vi "Perform Action.vi"(8 "error in":errorcluster, 10 "Input":variant, 11 "Red-y Read Write CFG in":refnum<class "Red-y Read Write CFG.lvclass">) -> (0 "error out":errorcluster, 2 "Output":variant, 3 "Red-y Read Write CFG out":refnum<class "Red-y Read Write CFG.lvclass">)   [LabVIEW 2023, in "Red-y Read Write CFG.lvclass"]
uses:
  Red-y Read Write CFG.lvclass
  Red-y Read Write CFG.lvclass/Red-y Read Write CFG.ctl
  Voegtlin_NI_SMART_Modbus_Drivers/Low Level Driver/Modbus Write U8.vi
  Voegtlin_NI_SMART_Modbus_Drivers/Low Level Driver/Modbus Write U16.vi
  Voegtlin_NI_SMART_Modbus_Drivers/Low Level Driver/Modbus Write U32.vi
  Voegtlin_NI_SMART_Modbus_Drivers/Low Level Driver/Modbus Write SGL.vi
  Voegtlin_NI_SMART_Modbus_Drivers/Low Level Driver/Modbus Write STR50.vi
  Voegtlin_NI_SMART_Modbus_Drivers/Low Level Driver/Modbus Read U8.vi
  Voegtlin_NI_SMART_Modbus_Drivers/Low Level Driver/Modbus Read U16.vi
  Voegtlin_NI_SMART_Modbus_Drivers/Low Level Driver/Modbus Read U32.vi
  Voegtlin_NI_SMART_Modbus_Drivers/Low Level Driver/Modbus Read SGL.vi
  Voegtlin_NI_SMART_Modbus_Drivers/Low Level Driver/Modbus Read STR50.vi
  <userlib>/_OpenG.lib/lvdata/lvdata.llb/openg_variant.lvlib
  Voegtlin_NI_SMART_Modbus_Drivers/Voegtlin_NI_SMART_Modbus_Drivers.lvlib
  Read Write PE Input.ctl
  <vilib>/ErrorRing/Error Ring.xnode
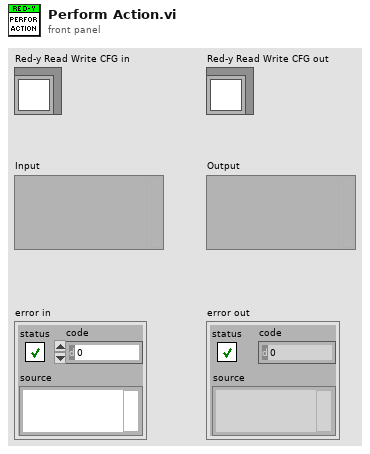
[diagram p1: front panel]
types:
  T1 = typedef "Read Write PE Input.ctl" = cluster{"Action":enum16{"Write", "Read"}, "Register Start Address":u16, "Data (Type)":variant}
  T2 = typedef "openg_variant.lvlib/Type Descriptor Enumeration__ogtk.ctl" = enum8{"<Null>", "I8", "I16", "I32", "I64", "U8", "U16", "U32", "U64", "SGL", "DBL", "EXT", "CSG", "CDB", "CXT", "0x0F", "0x10", "0x11", "0x12", "0x13", "0x14", "Enum U8", "Enum U16", "Enum U32", "Enum U64", "SGL PQ", "DBL PQ", "EXT PQ", "CSG PQ", "CDB PQ", "CXT PQ", "0x1F", "0x20", "Boolean", "0x22", "0x23", "0x24", "0x25", "0x26", "0x27", "0x28", "0x29", "0x2A", "0x2B", "0x2C", "0x2D", "0x2E", "0x2F", "String", "0x31", "Path", "Pict", "0x34", "0x35", "0x36", "DAQ", "0x38", "0x39", "0x3A", "0x3B", "0x3C", "0x3D", "0x3E", "0x3F", "Array", "0x41", "0x42", "0x43", "0x44", "0x45", "0x46", "0x47", "0x48", "0x49", "0x4A", "0x4B", "0x4C", "0x4D", "0x4E", "0x4F", "Cluster", "0x51", "0x52", "Variant", "Waveform", "0x55", "0x56", "0x57", "0x58", "0x59", "0x5A", "0x5B", "0x5C", "0x5D", "0x5E", "Fixed Point", "0x60", "0x61", "0x62", "0x63", "0x64", "0x65", "0x66", "0x67", "0x68", "0x69", "0x6A", "0x6B", "0x6C", "0x6D", "0x6E", "0x6F", "Refnum", "0x71", "0x72", "Set Collection", "Map Collection"}
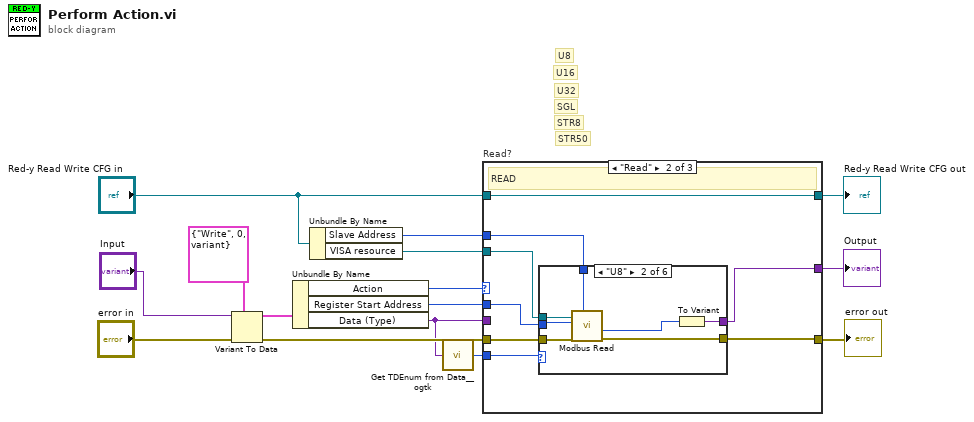
[diagram p0: block diagram]
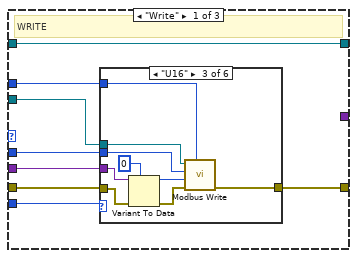
[diagram p2: hidden frame]
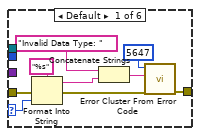
[diagram p3: hidden frame]
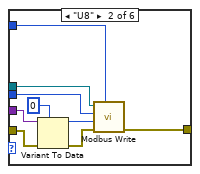
[diagram p4: hidden frame]
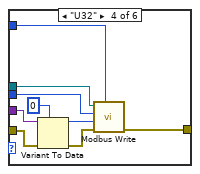
[diagram p5: hidden frame]
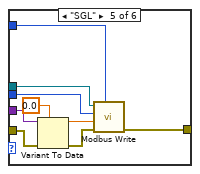
[diagram p6: hidden frame]
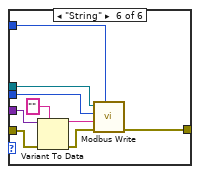
[diagram p7: hidden frame]
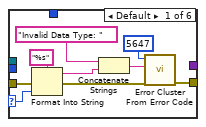
[diagram p8: hidden frame]
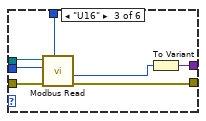
[diagram p9: hidden frame]
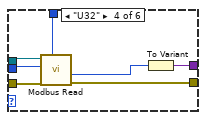
[diagram p10: hidden frame]
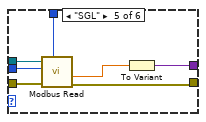
[diagram p11: hidden frame]
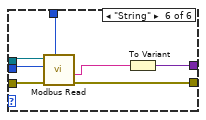
[diagram p12: hidden frame]
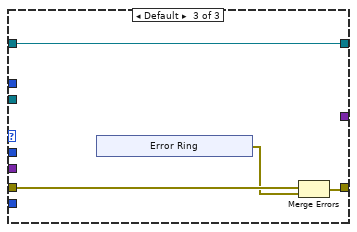
[diagram p13: hidden frame]
diagram:
  # "STR50"
  # "STR8"
  # "SGL"
  # "U32"
  # "U16"
  # "U8"
  n1 = Variant To Data(error in="error in", type=T1 {"Action"=enum."Write", "Register Start Address"=0, "Data (Type)"=variant}, Variant="Input") -> (data=w8:T1, error out=w11:errorcluster)
  n2 = Unbundle By Name(w8) -> ("Action"=w1:enum16{"Write", "Read"}, "Register Start Address"=w3:u16, "Data (Type)"=w2:variant)
  n3 = Unbundle By Name("Red-y Read Write CFG in") -> ("Slave Address"=w6:u8, "VISA resource"=w5:refnum<visa-resource-name>)
  n4 = call <userlib>:"Get TDEnum from Data__ogtk.vi"("Data"=w2) -> ("Type Descriptor Enumeration"=w4:T2)  [unwired: 4 in]
  n5 = case "Read?" shown="\"Read\"" w1 {
    tunnel: "Red-y Read Write CFG in" -> [w23 w85 w130]
    tunnel: [w23 w85 w130] -> w14
    tunnel: [w21 w82 w133] -> w13
    tunnel: w11 -> [w22 w84 w132]
    tunnel: [_ w83 _] -> w7
    tunnel: w6 -> [w19 w81 _]
    tunnel: w5 -> [w20 w80 _]
    tunnel: w4 -> [w17 w79 _]
    tunnel: w3 -> [w18 w78 _]
    tunnel: w2 -> [w16 _ _]
    frame "Write" {
      # "WRITE"
      n6 = case shown="\"U16\"" w17 {
        selector: w17 -> [w26 _ _ _ _ _]
        tunnel: w22 -> [w28 w37 w46 w55 w64 w73]
        tunnel: [w32 w41 w50 w59 w68 w77] -> w21
        tunnel: w20 -> [_ w40 w49 w58 w67 w76]
        tunnel: w19 -> [_ w39 w48 w57 w66 w75]
        tunnel: w18 -> [_ w38 w47 w56 w65 w74]
        tunnel: w16 -> [_ w35 w44 w53 w62 w71]
        frame Default {
          n7 = Format Into String(format string="%s", error in=w28, w26) -> (resulting string=w24:string, error out=w27:errorcluster)  [unwired: 1 in]
          n8 = Concatenate Strings("Invalid Data Type: ", w24) -> (w30:string)
          n9 = call <vilib>:"Error Cluster From Error Code.vi"("error in (no error)"=w27, "error message (\"\")"=w30, "error code (0)"=5647) -> ("error out"=w32:errorcluster)  [unwired: 6 in]
        }
        frame "U8" {
          n10 = Variant To Data(error in=w37, type=u8 0, Variant=w35) -> (data=w33:u8, error out=w36:errorcluster)
          n11 = call-poly "Modbus Write.vi"("Slave Address"=w39, "error in (no error)"=w36, "Input data U8"=w33, "Register Start Address"=w38, "VISA resource in"=w40) -> ("error out"=w41:errorcluster)  [unwired: 5 in, 1 out]
        }
        frame "U16" {
          n12 = Variant To Data(error in=w46, type=u16 0, Variant=w44) -> (data=w42:u16, error out=w45:errorcluster)
          n13 = call-poly "Modbus Write.vi"("Slave Address"=w48, "error in (no error)"=w45, "Input data U16"=w42, "Register Start Address"=w47, "VISA resource in"=w49) -> ("error out"=w50:errorcluster)  [unwired: 5 in, 1 out]
        }
        frame "U32" {
          n14 = Variant To Data(error in=w55, type=u32 0, Variant=w53) -> (data=w51:u32, error out=w54:errorcluster)
          n15 = call-poly "Modbus Write.vi"("Slave Address"=w57, "error in (no error)"=w54, "Input data U32"=w51, "Register Start Address"=w56, "VISA resource in"=w58) -> ("error out"=w59:errorcluster)  [unwired: 5 in, 1 out]
        }
        frame "SGL" {
          n16 = Variant To Data(error in=w64, type=sgl 0.0, Variant=w62) -> (data=w60:sgl, error out=w63:errorcluster)
          n17 = call-poly "Modbus Write.vi"("Slave Address"=w66, "error in (no error)"=w63, "Input data float32"=w60, "Register Start Address"=w65, "VISA resource in"=w67) -> ("error out"=w68:errorcluster)  [unwired: 5 in, 1 out]
        }
        frame "String" {
          n18 = Variant To Data(error in=w73, type="", Variant=w71) -> (data=w69:string, error out=w72:errorcluster)
          n19 = call-poly "Modbus Write.vi"("Slave Address"=w75, "error in (no error)"=w72, "Input String (50 chars)"=w69, "Register Start Address"=w74, "VISA resource in"=w76) -> ("error out"=w77:errorcluster)  [unwired: 5 in, 1 out]
        }
      }
    }
    frame "Read" {
      # "READ"
      n20 = case shown="\"U8\"" w79 {
        selector: w79 -> [w88 _ _ _ _ _]
        tunnel: w84 -> [w90 w101 w108 w115 w122 w126]
        tunnel: [w94 w100 w107 w114 w121 w124] -> w82
        tunnel: w81 -> [_ w99 w106 w113 w120 w129]
        tunnel: w80 -> [_ w95 w103 w111 w119 w127]
        tunnel: w78 -> [_ w98 w102 w112 w118 w128]
        tunnel: [_ w96 w105 w109 w116 w125] -> w83
        frame Default {
          n21 = Format Into String(format string="%s", error in=w90, w88) -> (resulting string=w86:string, error out=w89:errorcluster)  [unwired: 1 in]
          n22 = Concatenate Strings("Invalid Data Type: ", w86) -> (w92:string)
          n23 = call <vilib>:"Error Cluster From Error Code.vi"("error in (no error)"=w89, "error message (\"\")"=w92, "error code (0)"=5647) -> ("error out"=w94:errorcluster)  [unwired: 6 in]
        }
        frame "U8" {
          n24 = call-poly "Modbus Read.vi"("Slave Address"=w99, "error in (no error)"=w101, "Register Start Address"=w98, "VISA resource in"=w95) -> ("error out"=w100:errorcluster, "Output data U8"=w97:u8)  [unwired: 5 in, 1 out]
          n25 = To Variant(anything=w97) -> (Variant=w96:variant)
        }
        frame "U16" {
          n26 = call-poly "Modbus Read.vi"("Slave Address"=w106, "error in (no error)"=w108, "Register Start Address"=w102, "VISA resource in"=w103) -> ("error out"=w107:errorcluster, "Output data U16"=w104:u16)  [unwired: 5 in, 1 out]
          n27 = To Variant(anything=w104) -> (Variant=w105:variant)
        }
        frame "U32" {
          n28 = call-poly "Modbus Read.vi"("Slave Address"=w113, "error in (no error)"=w115, "Register Start Address"=w112, "VISA resource in"=w111) -> ("error out"=w114:errorcluster, "Output data U32"=w110:u32)  [unwired: 5 in, 1 out]
          n29 = To Variant(anything=w110) -> (Variant=w109:variant)
        }
        frame "SGL" {
          n30 = call-poly "Modbus Read.vi"("Slave Address"=w120, "error in (no error)"=w122, "Register Start Address"=w118, "VISA resource in"=w119) -> ("error out"=w121:errorcluster, "Output data float32"=w117:sgl)  [unwired: 5 in, 1 out]
          n31 = To Variant(anything=w117) -> (Variant=w116:variant)
        }
        frame "String" {
          n32 = call-poly "Modbus Read.vi"("Slave Address"=w129, "error in (no error)"=w126, "Register Start Address"=w128, "VISA resource in"=w127) -> ("error out"=w124:errorcluster, "Output string (50 chars)"=w123:string)  [unwired: 5 in, 1 out]
          n33 = To Variant(anything=w123) -> (Variant=w125:variant)
        }
      }
    }
    frame Default {
      n34 = xnode "Error Ring"() -> ("error out"=w131:errorcluster)
      n35 = Merge Errors(w132, w131) -> (w133:errorcluster)
    }
  }
  "error out" <- w13
  "Red-y Read Write CFG out" <- w14
  "Output" <- w7
